vi "ChemicalTank.vi"(4 "Capacity (mB)":i64, 5 "Last Fill (mB)":i64, 8 "Transfer (mB)":i64) -> (0 "Fill (mB)":i64, 1 "Needed (mB)":i64, 2 "Overflow":bool, 3 "Overflow (mB)":i64)   [LabVIEW 2024]
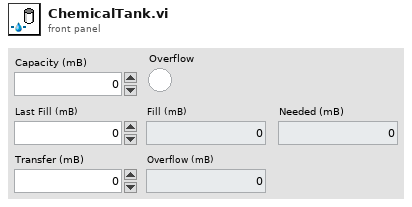
[diagram p1: front panel]
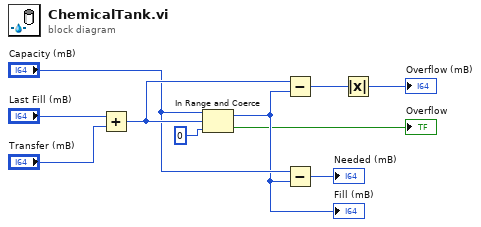
[diagram p0: block diagram]
diagram:
  n1 = Add(x="Last Fill (mB)", y="Transfer (mB)") -> (x+y=w7:i64)
  n2 = In Range and Coerce(upper limit="Capacity (mB)", x=w7, lower limit=i64 0) -> (coerced(x)=w4:i64, In Range?=→"Overflow":bool)
  "Fill (mB)" <- w4
  n3 = Subtract(x=w7, y=w4) -> (x-y=w6:i64)
  n4 = Subtract(x="Capacity (mB)", y=w4) -> (x-y=→"Needed (mB)":i64)
  n5 = Absolute Value(x=w6) -> (abs(x)=→"Overflow (mB)":i64)
